vi "add_to_value-history.vi"(8 "error in (no error)":errorcluster, 10 "Cluster":cluster{"time as number":dbl, "Value":dbl} {"time as number" format="%<%H:%M:%S\n%m/%d/%y>T"}, 11 "PrepLineObject in":refnum<class "PrepLineObject.lvclass">) -> (0 "error out":errorcluster, 3 "PrepLineObject out":refnum<class "PrepLineObject.lvclass">)   [LabVIEW 2018, in "PrepLineObject.lvclass"]
doc: "adds a value to the value-history array. The history array is a private property"
uses:
  PrepLineObject.lvclass
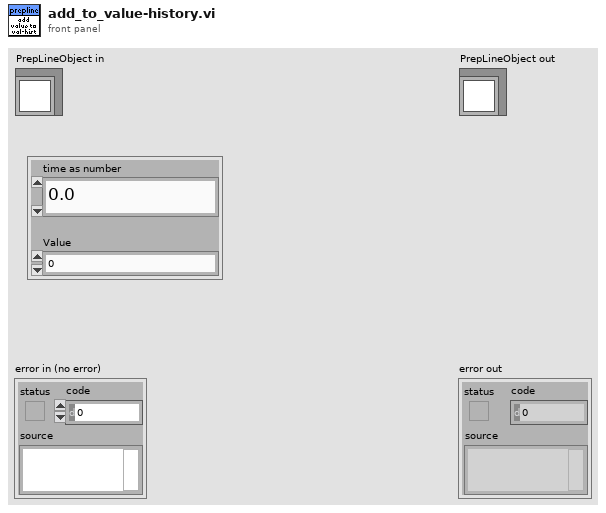
[diagram p1: front panel]
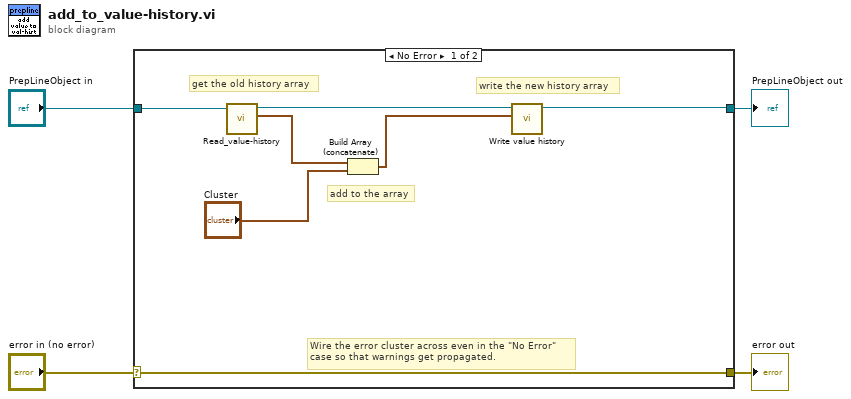
[diagram p0: block diagram]
diagram:
  n1 = case shown="No Error" "error in (no error)" {
    selector: "error in (no error)" -> [w11 w13]
    tunnel: [w11 w13] -> w3
    tunnel: [w8 w12] -> w1
    tunnel: "PrepLineObject in" -> [w10 w12]
    frame No Error {
      # "write the new history array"
      # "add to the array"
      # "get the old history array"
      # "Wire the error cluster across even in the \"No Error\"\ncase so that warnings get propagated."
      n2 = call-dynamic "Read_value-history.vi"("PrepLineObject in"=w10) -> ("value history"=w7:cluster{"time as number":dbl, "Value":dbl}[], "PrepLineObject out"=w9:refnum<class "PrepLineObject.lvclass">)  [unwired: 8 in, 1 out]
      n3 = Build Array (concatenate)(w7, "Cluster") -> (w6:cluster{"time as number":dbl, "Value":dbl}[])
      n4 = call-dynamic "Write value history.vi"("value history"=w6, "PrepLineObject in"=w9) -> ("PrepLineObject out"=w8:refnum<class "PrepLineObject.lvclass">)  [unwired: 8 in, 1 out]
    }
    frame Error {
    }
  }
  "error out" <- w3
  "PrepLineObject out" <- w1
